vi "puls_generator_control.VI"() -> ()   [LabVIEW 2015]
panel:
  in  "DO8":u16
  in  "TO8":u16
  in  "D02":u16=100
  in  "Send O CTRL":bool
  in  "TM0H":u16
  in  "TM0L":u16=1000
  in  "DO7":u16
  in  "TO7":u16
  in  "DO6":u16
  in  "TO6":u16
  in  "DO5":u16
  in  "TO5":u16
  in  "DO4":u16
  in  "T04":u16
  in  "DO3":u16
  in  "TO3":u16
  in  "TO2":u16=10
  # "Tn: delay"
  # "Dn: duration"
  # "*5ns"
  # "TO1: T0 main clock"
  # "period"
  # "*10ns"
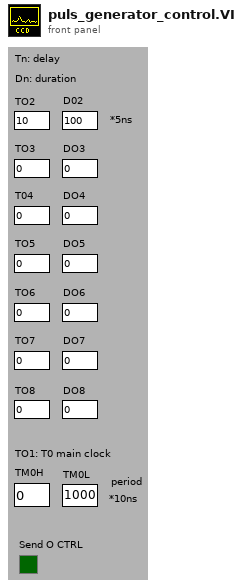
[diagram p1: front panel]
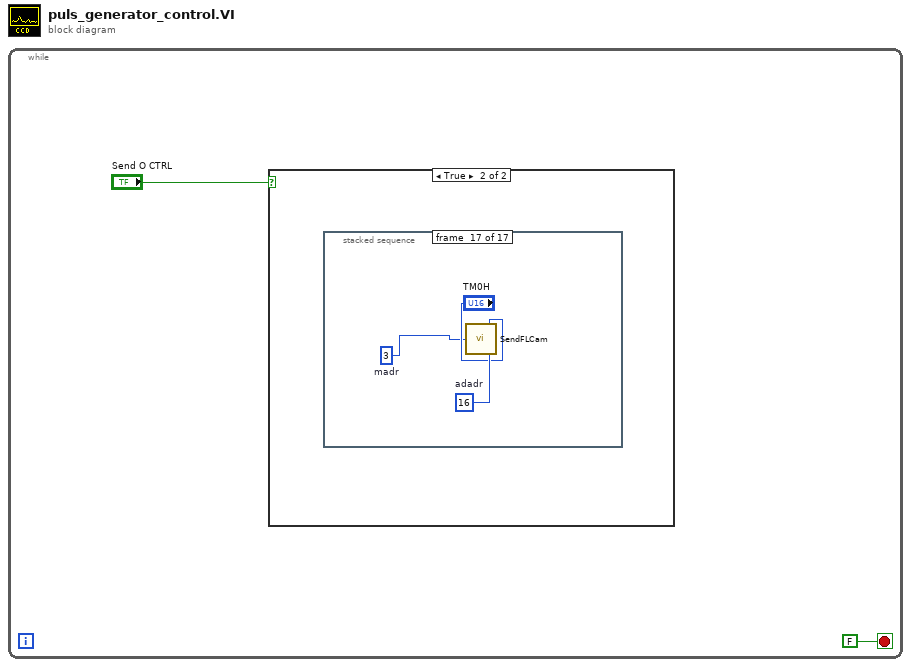
[diagram p0: block diagram]
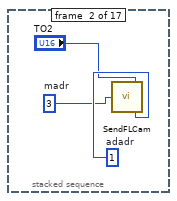
[diagram p4: hidden frame]
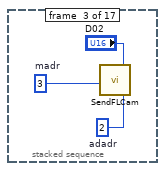
[diagram p5: hidden frame]
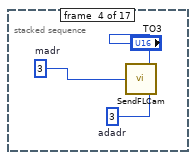
[diagram p6: hidden frame]
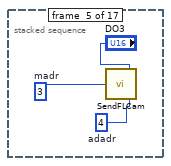
[diagram p7: hidden frame]
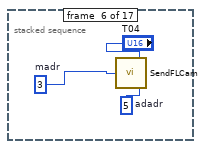
[diagram p8: hidden frame]
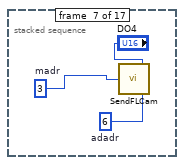
[diagram p9: hidden frame]
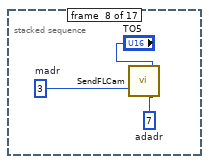
[diagram p10: hidden frame]
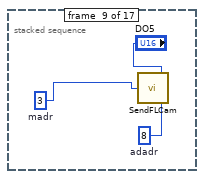
[diagram p11: hidden frame]
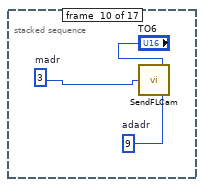
[diagram p12: hidden frame]
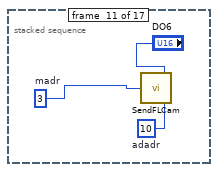
[diagram p13: hidden frame]
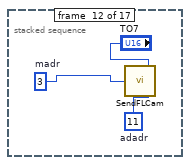
[diagram p14: hidden frame]
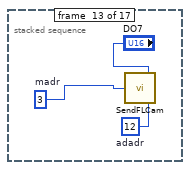
[diagram p15: hidden frame]
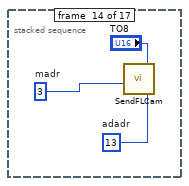
[diagram p16: hidden frame]
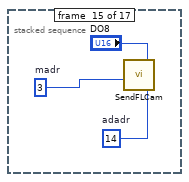
[diagram p17: hidden frame]
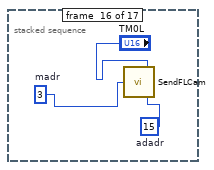
[diagram p18: hidden frame]
diagram:
  n1 = while {
    stop <- FALSE stop-if-true
    n2 = case shown="True" "Send O CTRL" {
      frame False {
      }
      frame True {
        n3 = stacked-sequence {
          frame #0 {
          }
          frame #1 {
            w5 = 1  # adadr
            w4 = 3  # madr
            n4 = call "SendFLCam.vi"("madr"=w4, "data"="TO2", "adadr"=w5) -> ()
          }
          frame #2 {
            w7 = 2  # adadr
            w8 = 3  # madr
            n5 = call "SendFLCam.vi"("madr"=w8, "data"="D02", "adadr"=w7) -> ()
          }
          frame #3 {
            w11 = 3  # adadr
            w10 = 3  # madr
            n6 = call "SendFLCam.vi"("madr"=w10, "data"="TO3", "adadr"=w11) -> ()
          }
          frame #4 {
            w14 = 4  # adadr
            w13 = 3  # madr
            n7 = call "SendFLCam.vi"("madr"=w13, "data"="DO3", "adadr"=w14) -> ()
          }
          frame #5 {
            w17 = 5  # adadr
            w16 = 3  # madr
            n8 = call "SendFLCam.vi"("madr"=w16, "data"="T04", "adadr"=w17) -> ()
          }
          frame #6 {
            w20 = 6  # adadr
            w19 = 3  # madr
            n9 = call "SendFLCam.vi"("madr"=w19, "data"="DO4", "adadr"=w20) -> ()
          }
          frame #7 {
            w23 = 7  # adadr
            w22 = 3  # madr
            n10 = call "SendFLCam.vi"("madr"=w22, "data"="TO5", "adadr"=w23) -> ()
          }
          frame #8 {
            w26 = 8  # adadr
            w25 = 3  # madr
            n11 = call "SendFLCam.vi"("madr"=w25, "data"="DO5", "adadr"=w26) -> ()
          }
          frame #9 {
            w27 = 9  # adadr
            w29 = 3  # madr
            n12 = call "SendFLCam.vi"("madr"=w29, "data"="TO6", "adadr"=w27) -> ()
          }
          frame #10 {
            w32 = 10  # adadr
            w31 = 3  # madr
            n13 = call "SendFLCam.vi"("madr"=w31, "data"="DO6", "adadr"=w32) -> ()
          }
          frame #11 {
            w35 = 11  # adadr
            w34 = 3  # madr
            n14 = call "SendFLCam.vi"("madr"=w34, "data"="TO7", "adadr"=w35) -> ()
          }
          frame #12 {
            w38 = 12  # adadr
            w37 = 3  # madr
            n15 = call "SendFLCam.vi"("madr"=w37, "data"="DO7", "adadr"=w38) -> ()
          }
          frame #13 {
            w40 = 13  # adadr
            w41 = 3  # madr
            n16 = call "SendFLCam.vi"("madr"=w41, "data"="TO8", "adadr"=w40) -> ()
          }
          frame #14 {
            w43 = 14  # adadr
            w44 = 3  # madr
            n17 = call "SendFLCam.vi"("madr"=w44, "data"="DO8", "adadr"=w43) -> ()
          }
          frame #15 {
            w46 = 15  # adadr
            w47 = 3  # madr
            n18 = call "SendFLCam.vi"("madr"=w47, "data"="TM0L", "adadr"=w46) -> ()
          }
          frame #16 {
            w50 = 16  # adadr
            w48 = 3  # madr
            n19 = call "SendFLCam.vi"("madr"=w48, "data"="TM0H", "adadr"=w50) -> ()
          }
        }
      }
    }
  }
